vi "Nested Parameterized.vi"   [LabVIEW 2020, in "Caraya Extension Tests.lvclass"]
uses:
  Caraya Extension Tests.lvclass
  <vilib>/addons/_JKI Toolkits/Caraya/classes/Test/Test.lvclass
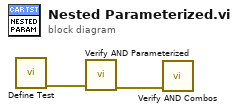
[diagram p0: block diagram]
diagram:
  n1 = call <vilib>:"Define Test.vi"() -> ("error out"=w1:errorcluster)  [unwired: 10 in, 1 out]
  n2 = call "Verify AND Parameterized.vi"("error in"=w1) -> ("error out"=w2:errorcluster)  [unwired: 10 in]
  n3 = call "Verify AND Combos.vi"("error in"=w2) -> ()  [unwired: 10 in, 1 out]
